vi "00 - Simple Debugging.vi"() -> ()   [LabVIEW 2025]
uses:
  <vilib>/Utility/file.llb/Write Delimited Spreadsheet (DBL).vi
  <vilib>/Utility/sysdir.llb/System Directory Type.ctl
panel:
  out "Array 2":path[](array[path])
  out "Array":T1(array[cluster])
  # "Open Block Diagram to Debug Code\nCtl + E (instructions on diagram)"
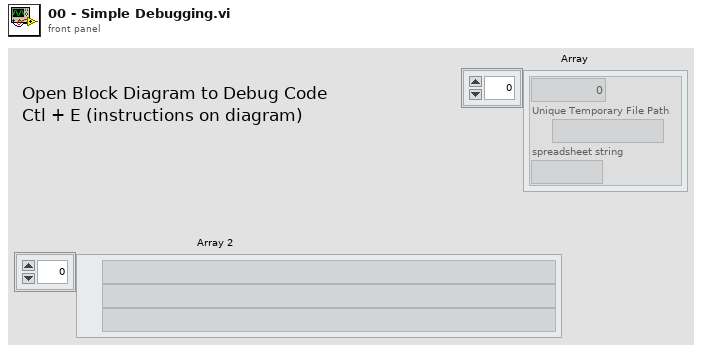
[diagram p1: front panel]
types:
  T1 = cluster{"Numeric":i32, "Unique Temporary File Path":path, "spreadsheet string":string}[]
  T2 = typedef "System Directory Type.ctl" = i32
  T3 = cluster{i32, "Unique Temporary File Path":path, "spreadsheet string":string}
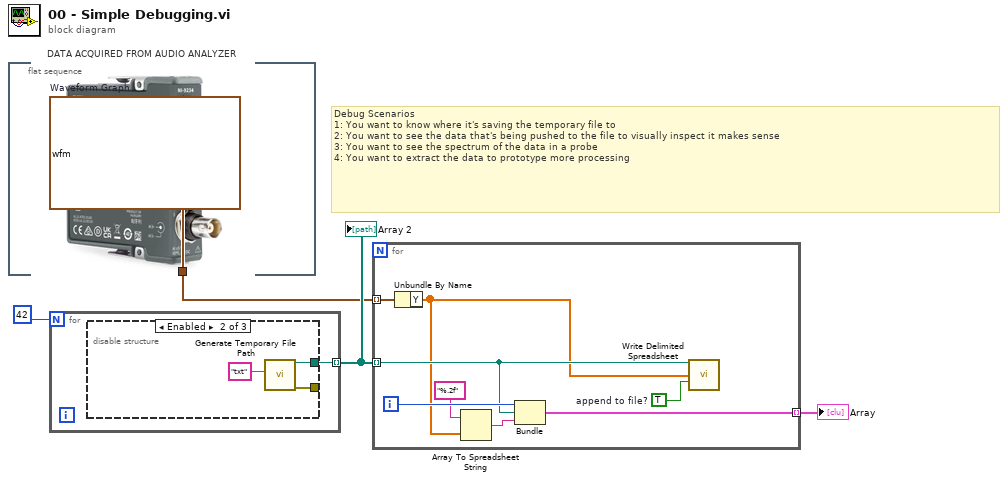
[diagram p0: block diagram]
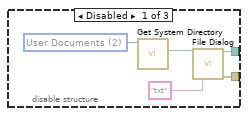
[diagram p2: hidden frame]
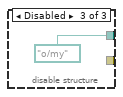
[diagram p3: hidden frame]
diagram:
  # "Debug Scenarios\n1: You want to know where it's saving the temporary file to\n2: You want to see the data that's being pushed to the file to visually inspect it makes sense\n3: You want to see the spectrum of the data in a probe\n4: You want to extract the data to prototype more processing"
  n1 = flat-sequence "DATA ACQUIRED FROM AUDIO ANALYZER" {
    tunnel: [w5] -> w3
    frame #0 {
      w5 = waveform(dbl)[] [{"t0"=timestamp(0 s since 1904-01-01), "dt"=0.0002, "Y"=array[5000 elements]}, {"t0"=timestamp(0 s since 1904-01-01), "dt"=0.0002, "Y"=array[5000 elements]}]  # Waveform Graph
    }
  }
  n2 = for {
    N: 42 -> [_]
    tunnel: [w6] -> w4 mode=indexing
    n3 = disable-structure shown="Enabled" {
      disable-tunnel: [w11 w14 _] -> _
      disable-tunnel: [w8 w12 path "o:/my" ("selected path")] -> w6
      frame Disabled {
        w9 = T2 2 items=["User Home"=0, "User Desktop"=1, "User Documents"=2, "User Application Data"=3, "User Preferences"=4, "User Temporary"=5, "Public Documents"=6, "Public Application Data"=7, "Public Preferences"=8, "Public Cache"=13, "System Core Libraries"=9, "System Installed Libraries"=10, "Application Files"=11, "Boot Volume Root"=12] ("system directory type")
        n4 = call <vilib>:"Get System Directory.vi"("system directory type"=w9) -> ("system directory"=w10:path)  [unwired: 10 in]
        n5 = call "File Dialog"("start path"=w10, "pattern (all files)"="txt") -> ("selected path"=w8:path, "error out"=w11:errorcluster)  [unwired: 10 in, 2 out]
      }
      frame Enabled {
        n6 = call <vilib>:"Generate Temporary File Path.vi"("Temporary File Extension (tmp)"="txt" ("pattern (all files)")) -> ("error out"=w14:errorcluster, "Unique Temporary File Path"=w12:path)  [unwired: 9 in]
      }
      frame Disabled {
      }
    }
  }
  "Array 2" <- w4
  n7 = for {
    tunnel: w3 -> [w22] mode=indexing
    tunnel: w4 -> [w20] mode=indexing
    tunnel: [w18] -> w2 mode=indexing
    i -> [w21]
    w23 = TRUE  # append to file?
    n8 = Unbundle By Name(w22) -> ("Y"=w19:dbl[])
    n9 = Array To Spreadsheet String(array=w19, 3:"%.2f" ("format string")) -> (spreadsheet string=w16:string)  [unwired: 1 in]
    n10 = Bundle(w21, "Unique Temporary File Path"=w20, "spreadsheet string"=w16) -> (w18:T3)  [unwired: 1 in]
    n11 = call-poly <vilib>:"Write Delimited Spreadsheet.vi"("file path (dialog if empty)"=w20, "1D data"=w19, "append to file? (new file:F)"=w23) -> ()  [unwired: 11 in, 2 out]
  }
  "Array" <- w2
